vi "Add Character to Content.vi"(8 "Error In":errorcluster, 10 "Character":u8, 11 "Parser In":refnum<class "Parser.lvclass">) -> (0 "Error Out":errorcluster, 3 "Parser Out":refnum<class "Parser.lvclass">)   [LabVIEW 2017, in "Mustache.lvlib" / "Parser.lvclass"]
uses:
  Parser.lvclass
  Parser.lvclass/Parser.ctl
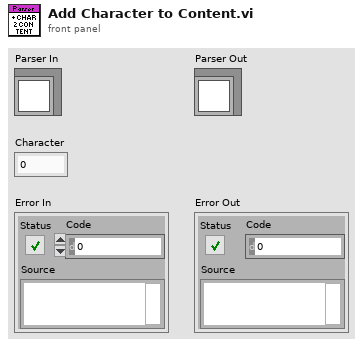
[diagram p1: front panel]
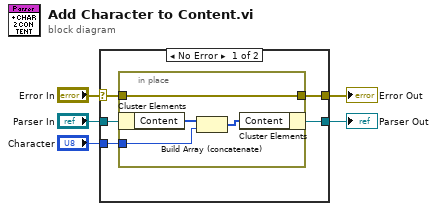
[diagram p0: block diagram]
diagram:
  n1 = case shown="No Error" "Error In" {
    selector: "Error In" -> [w6 w15]
    tunnel: [w10 w15] -> w5
    tunnel: "Character" -> [w9 _]
    tunnel: [w8 w16] -> w3
    tunnel: "Parser In" -> [w7 w16]
    frame No Error {
      n2 = in-place {
        in-place-border: w9 -> [w13]
        in-place-border: w6 -> [w11]
        in-place-border: [w11] -> w10
        n3 = in-place-cluster #1(w7) -> ("Content"=w14:u8[])
        n4 = Build Array (concatenate)(w14, w13) -> (w12:u8[])
        n5 = in-place-cluster #1("Content"=w12) -> (w8:refnum<class "Parser.lvclass">)
      }
    }
    frame Error {
    }
  }
  "Error Out" <- w5
  "Parser Out" <- w3
